vi "2023 Input Arm To Wrist Global.vi"() -> ()   [LabVIEW 2020]
panel:
  out "inputToArmToWristConversion":dbl[](array[numeric])
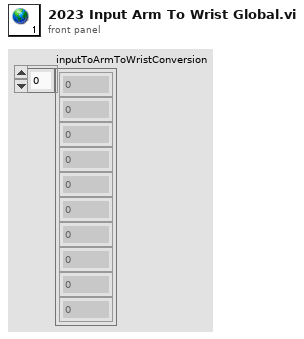
[diagram p1: front panel]
diagram:
